vi "get app name.vi"(7 "Current VI's Path":path) -> (1 "Is EXE?":bool, 2 "App Name Without Extension":string, 3 "App Name":string)   [LabVIEW 2021]
doc: "Checks the current path to this VI to see if it is called as part of an executable. If so, the \"Quit LabVIEW\" VI is called.\n\nsupport@labjack.com\nwww.labjack.com\n6/17/2001"
panel:
  # "If running a source VI, \"Current VI's Path\" returns something like:\n\nC:\\Users\\Toby\\SkyDrive\\hostapp\\LabVIEW\\LabVIEW_LJUD\\Examples\\LJLogUD\\LJLogUD.vi\n\n... and this VI will return \"LJLogUD.vi\".  If running an exe, \"Current VI's Path\" returns something like:\n\nC:\\temp\\LJLogUD_build\\LJLogUD.exe\\LJLogUD.vi"
  # "Pass in the output of \"Current VI's Path\", which can be found in Functions Palette => File I/O => File Constants."
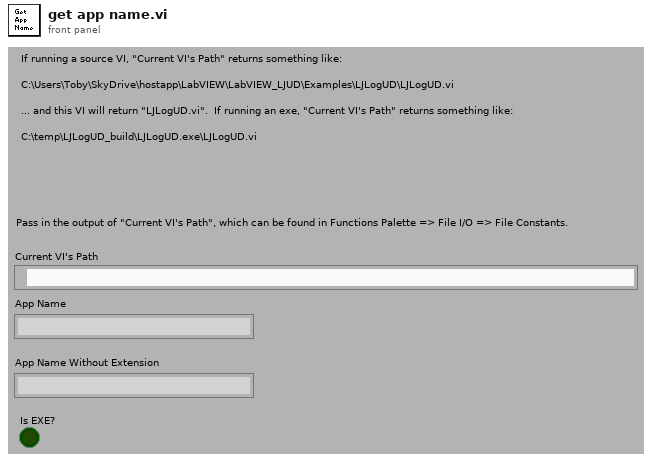
[diagram p1: front panel]
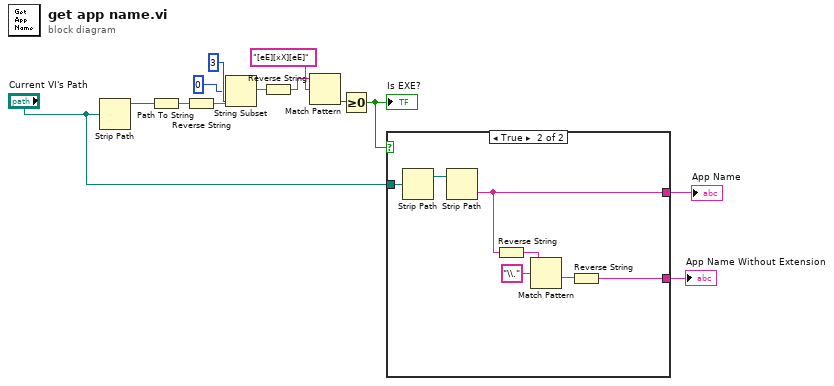
[diagram p0: block diagram]
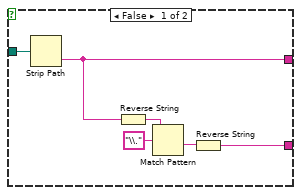
[diagram p2: hidden frame]
diagram:
  n1 = Strip Path(path="Current VI's Path") -> (stripped path=w5:path)  [unwired: 1 out]
  n2 = Path To String(path=w5) -> (string=w13:string)
  n3 = Reverse String(1:w13) -> (0:w12:string)
  n4 = String Subset(string=w12, offset (0)=0, length (rest)=3 ("length")) -> (substring=w9:string)
  n5 = Reverse String(1:w9) -> (0:w8:string)
  n6 = Match Pattern(string=w8, regular expression="[eE][xX][eE]") -> (offset past match=w6:i32)  [unwired: 1 in, 3 out]
  n7 = Greater Or Equal To 0?(x=w6) -> (x >= 0?=w4:bool)
  "Is EXE?" <- w4
  n8 = case shown="True" w4 {
    tunnel: "Current VI's Path" -> [w16 w23]
    tunnel: [w15 w20] -> w2
    tunnel: [w14 w22] -> w1
    frame False {
      n9 = Strip Path(path=w16) -> (name=w15:string)  [unwired: 1 out]
      n10 = Reverse String(1:w15) -> (0:w18:string)
      n11 = Match Pattern(string=w18, regular expression="\\.") -> (after substring=w17:string)  [unwired: 1 in, 3 out]
      n12 = Reverse String(1:w17) -> (0:w14:string)
    }
    frame True {
      n13 = Strip Path(path=w23) -> (stripped path=w21:path)  [unwired: 1 out]
      n14 = Strip Path(path=w21) -> (name=w20:string)  [unwired: 1 out]
      n15 = Reverse String(1:w20) -> (0:w25:string)
      n16 = Match Pattern(string=w25, regular expression="\\.") -> (after substring=w24:string)  [unwired: 1 in, 3 out]
      n17 = Reverse String(1:w24) -> (0:w22:string)
    }
  }
  "App Name" <- w2
  "App Name Without Extension" <- w1
